vi "Test SubPanel.vi"() -> ()   [LabVIEW 2010]
panel:
  in  "停止":bool
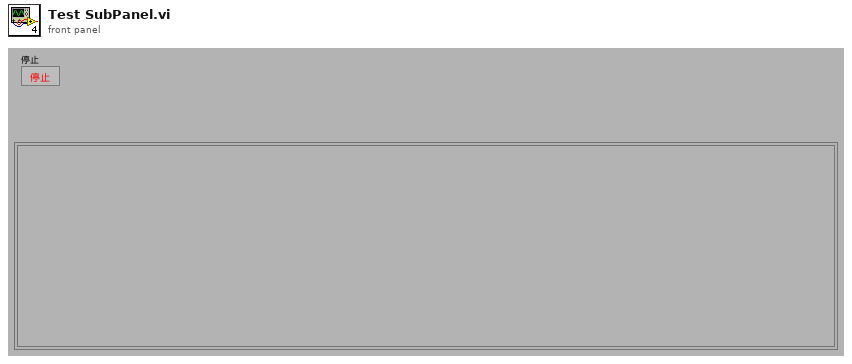
[diagram p1: front panel]
types:
  T1 = enum32{"Ramp", "Hold", "Loop", "Start", "Stop", "Idle"}
  T2 = typedef "Path InitDynamicVIsPaths__FS.ctl" = cluster{"F4 Operation":path, "F4 Alarms":path, "F4 Inputs":path, "F4 Outputs":path, "F4 PID Sets":path, "F4 Cascade":path, "F4 Current Step":path, "Profile SubPanel":path, "Profile Editor":path, "MainVI":path, "Profile Control":path, "Synergy Control":path, "Driver Server":path}
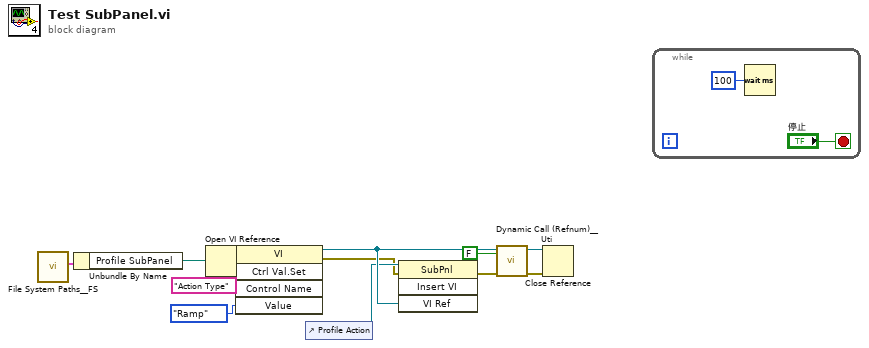
[diagram p0: block diagram]
diagram:
  n1 = call "File System Paths__FS.vi"() -> ("DynamicVIs"=w2:T2)  [unwired: 9 in, 2 out]
  n2 = Unbundle By Name(w2) -> ("Profile SubPanel"=w12:path)
  n3 = Open VI Reference(vi path=w12) -> (vi reference=w10:refnum<vi>)  [unwired: 5 in, 1 out]
  n4 = invoke class="VI" method="Ctrl Val.Set"(reference=w10, "Control Name"="Action Type" ("控件名"), "Value"=T1."Ramp" ("Action Type")) -> (reference out=w5:refnum<vi>, error out=w3:errorcluster)  [unwired: 2 in, 3 out]
  n5 = control-ref of="Profile Action"() -> (w4:refnum<vi>)
  n6 = invoke on="调用节点" class="SubPnl" method="Insert VI"(reference=w4, error in=w3, "VI Ref"=w5) -> (error out=w7:errorcluster)  [unwired: 1 in, 3 out]
  n7 = call "Dynamic Call (Refnum)__Uti.vi"("error in (no error)"=w7, "open front panel? (T)"=FALSE, "vi reference in"=w5) -> ("error out"=w9:errorcluster, "vi reference out"=w8:refnum<vi>)  [unwired: 7 in]
  n8 = Close Reference(reference=w8, error in (no error)=w9) -> ()  [unwired: 1 out]
  n9 = while {
    stop <- "停止" stop-if-true
    n10 = Wait (ms)(milliseconds to wait=u32 100 ("等待时间（毫秒）")) -> ()  [unwired: 1 out]
  }
